vi "Factorial To the Fourth.vi"(1 "N":i32) -> (0 "(N!)^4":T1={"Array Num"=[1, 2, 3], "Decimal Index"=0, "stop"=FALSE})   [LabVIEW 2025]
uses:
  Number.ctl
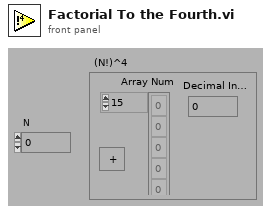
[diagram p1: front panel]
types:
  T1 = typedef "Number.ctl" = cluster{"Array Num":i8[], "Decimal Index":i32, "stop":bool}
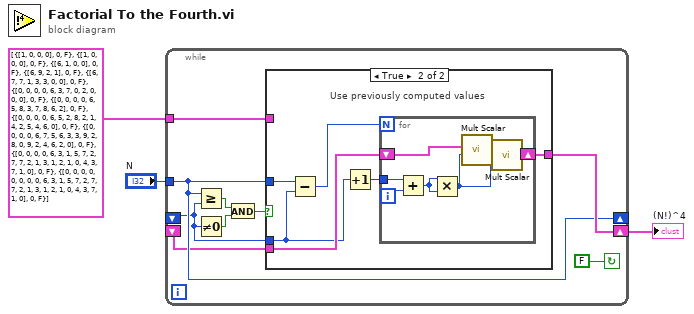
[diagram p0: block diagram]
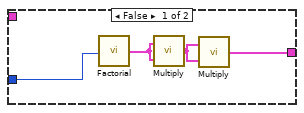
[diagram p2: hidden frame]
diagram:
  n1 = while {
    tunnel: "N" -> [w9]
    tunnel: T1[] [{"Array Num"=[1, 0, 0, 0], "Decimal Index"=0, "stop"=FALSE}, {"Array Num"=[1, 0, 0, 0], "Decimal Index"=0, "stop"=FALSE}, {"Array Num"=[6, 1, 0, 0], "Decimal Index"=0, "stop"=FALSE}, {"Array Num"=[6, 9, 2, 1], "Decimal Index"=0, "stop"=FALSE}, {"Array Num"=[6, 7, 7, 1, 3, 3, 0, 0], "Decimal Index"=0, "stop"=FALSE}, {"Array Num"=[0, 0, 0, 0, 6, 3, 7, 0, 2, 0, 0, 0], "Decimal Index"=0, "stop"=FALSE}, {"Array Num"=[0, 0, 0, 0, 6, 5, 8, 3, 7, 8, 6, 2], "Decimal Index"=0, "stop"=FALSE}, {"Array Num"=[0, 0, 0, 0, 6, 5, 2, 8, 2, 1, 4, 2, 5, 4, 6, 0], "Decimal Index"=0, "stop"=FALSE}, {"Array Num"=[0, 0, 0, 0, 6, 7, 5, 6, 3, 3, 9, 2, 8, 0, 9, 2, 4, 6, 2, 0], "Decimal Index"=0, "stop"=FALSE}, {"Array Num"=[0, 0, 0, 0, 6, 3, 1, 5, 7, 2, 7, 7, 2, 1, 3, 1, 2, 1, 0, 4, 3, 7, 1, 0], "Decimal Index"=0, "stop"=FALSE}, {"Array Num"=[0, 0, 0, 0, 0, 0, 0, 0, 6, 3, 1, 5, 7, 2, 7, 7, 2, 1, 3, 1, 2, 1, 0, 4, 3, 7, 1, 0], "Decimal Index"=0, "stop"=FALSE}] ("Array") -> [w12]
    shift-right: [w9] -> _
    shift-left: _ -> [w7]
    shift-right: [w10] -> w1
    shift-left: _ -> [w8]
    stop <- FALSE continue-if-true
    n2 = Greater Or Equal?(x=w9, y=w7) -> (x >= y?=w5:bool)
    n3 = Not Equal To 0?(x=w7) -> (x != 0?=w4:bool)
    n4 = And(x=w5, y=w4) -> (x .and. y?=w6:bool)
    n5 = case shown="True" w6 {
      tunnel: w12 -> [_ _]
      tunnel: [w13 w21] -> w10
      tunnel: w9 -> [w14 w20]
      tunnel: w8 -> [_ w22]
      tunnel: w7 -> [_ w18]
      frame False {
        n6 = call "Factorial.vi"("N"=w14) -> ("N!"=w15:T1)
        n7 = call "Multiply.vi"("B"=w15, "A"=w15) -> ("Answer"=w16:T1)
        n8 = call "Multiply.vi"("B"=w16, "A"=w16) -> ("Answer"=w13:T1)
      }
      frame True {
        # "Use previously computed values"
        n9 = Subtract(x=w20, y=w18) -> (x-y=w19:i32)
        n10 = Increment(x=w18) -> (x+1=w17:i32)
        n11 = for {
          N: w19 -> [_]
          tunnel: w17 -> [w29]
          shift-right: [w24] -> w21
          shift-left: w22 -> [w27]
          i -> [w28]
          n12 = Add(x=w29, y=w28) -> (x+y=w26:i32)
          n13 = Multiply(x=w26, y=w26) -> (x*y=w23:i32)
          n14 = call "Mult Scalar.vi"("A"=w27, "Scalar"=w23) -> ("A x Scalar"=w25:T1)  [unwired: 3 in]
          n15 = call "Mult Scalar.vi"("A"=w25, "Scalar"=w23) -> ("A x Scalar"=w24:T1)  [unwired: 3 in]
        }
      }
    }
  }
  "(N!)^4" <- w1
